vi "AMFreqminduration.vi"(4 "Offset":u8 max=0 step=1, 6 "Amplitude (%)":u8=32 min=1 max=100 step=1, 8 "Reps":u16=1, 10 "AM Freq (Hz)":dbl, 11 "LUT size":u8=32) -> (0 "Duration (ms)":dbl, 2 "AMout":string, 3 "Actual Freq":dbl)   [LabVIEW 2013]
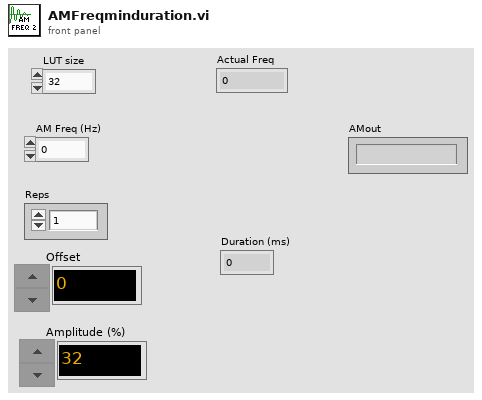
[diagram p1: front panel]
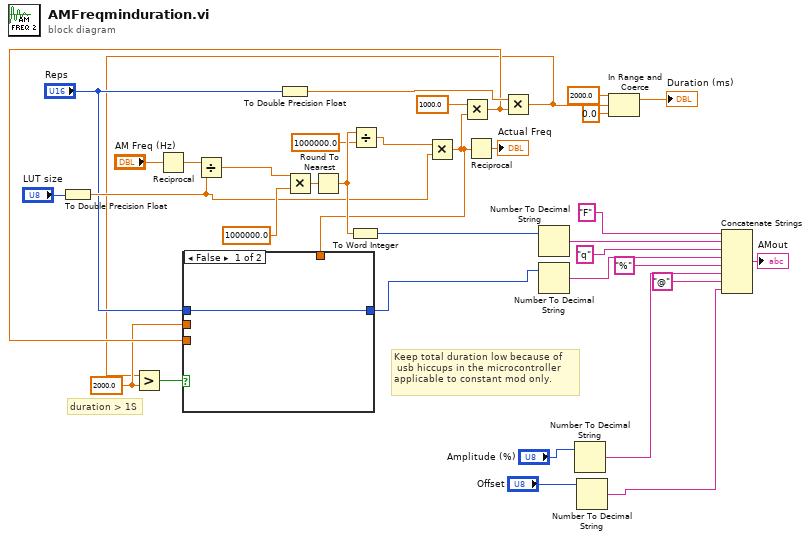
[diagram p0: block diagram]
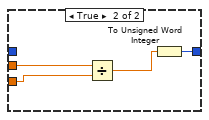
[diagram p2: hidden frame]
diagram:
  w5 = 2000.0 ("y")
  # "Keep total duration low because of\n usb hiccups in the microcontroller\napplicable to constant mod only."
  # "duration > 1S"
  n1 = To Double Precision Float(number="LUT size") -> (double precision float=w24:dbl)
  n2 = Reciprocal(x="AM Freq (Hz)") -> (1/x=w34:dbl)
  n3 = Divide(x=w34, y=w24) -> (x/y=w10:dbl)
  n4 = To Double Precision Float(number="Reps") -> (double precision float=w26:dbl)
  n5 = Multiply(x=w10, y=1000000.0) -> (x*y=w29:dbl)
  n6 = Round To Nearest(number=w29) -> (nearest integer value=w32:dbl)
  n7 = To Word Integer(number=w32) -> (16bit integer=w21:i16)
  n8 = Divide(x=w32, y=1000000.0) -> (x/y=w9:dbl)
  n9 = Multiply(x=w9, y=w24) -> (x*y=w7:dbl)
  n10 = Multiply(x=1000.0, y=w7) -> (x*y=w6:dbl)
  n11 = Reciprocal(x=w7) -> (1/x=→"Actual Freq":dbl)
  n12 = Multiply(x=w26, y=w6) -> (x*y=w4:dbl)
  n13 = Greater?(x=w4, y=w5) -> (0:w28:bool)
  n14 = case shown="False" w28 {
    tunnel: [w36 w40] -> w8
    tunnel: "Reps" -> [w36 _]
    tunnel: w7 -> [_ _]
    tunnel: w6 -> [_ w38]
    tunnel: w5 -> [_ w39]
    frame False {
    }
    frame True {
      n15 = Divide(x=w39, y=w38) -> (x/y=w37:dbl)
      n16 = To Unsigned Word Integer(number=w37) -> (unsigned 16bit integer=w40:u16)
    }
  }
  n17 = Number To Decimal String(number=w21) -> (decimal integer string=w22:string)  [unwired: 1 in]
  n18 = Number To Decimal String(number=w8) -> (decimal integer string=w19:string)  [unwired: 1 in]
  n19 = Number To Decimal String(number="Amplitude (%)") -> (decimal integer string=w15:string)  [unwired: 1 in]
  n20 = Number To Decimal String(number="Offset") -> (decimal integer string=w12:string)  [unwired: 1 in]
  n21 = In Range and Coerce(upper limit=2000.0, x=w4, lower limit=0.0) -> (coerced(x)=→"Duration (ms)":dbl)  [unwired: 1 out]
  n22 = Concatenate Strings("F" ("element"), w22, "q" ("string"), w19, "%" ("string"), w15, "@" ("string"), w12) -> (→"AMout":string)
